vi "Create-server-channel.vi"(8 "error in (no error)":errorcluster, 11 "ModComm in":T1) -> (0 "error out":errorcluster, 2 "ServerChannel":refnum<queue>, 3 "ModComm out":T1)   [LabVIEW 2013, in "SLMServer.lvlib" / "SLMServer.lvclass"]
uses:
  SLMServer.lvclass
  Object-reference.ctl
  SA-SLMAPI/Sources/Message.lvclass
  SLMServer.lvclass/SLMServer.ctl
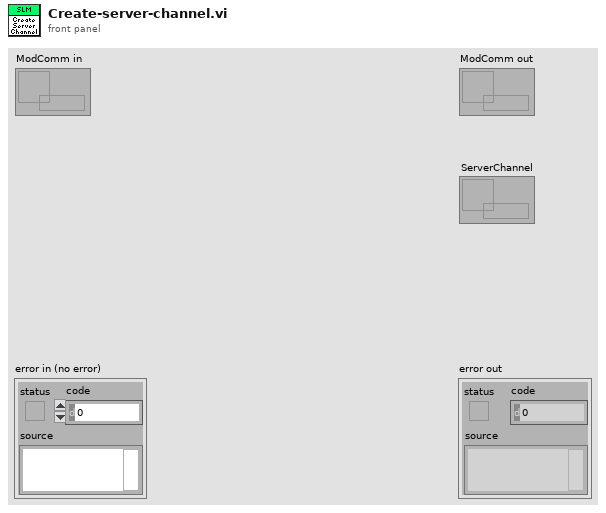
[diagram p1: front panel]
types:
  T1 = typedef "SLMServer.lvlib/SLMServer.lvclass/Object-reference.ctl" = refnum<data-value>
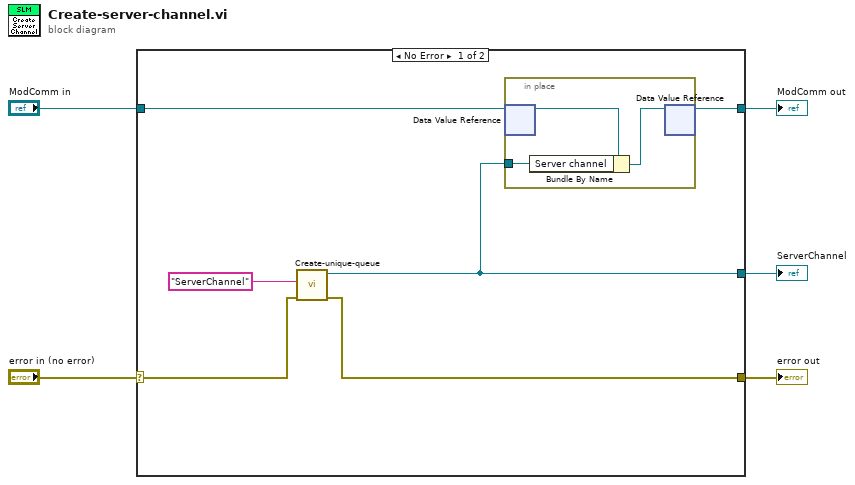
[diagram p0: block diagram]
diagram:
  n1 = case shown="No Error" "error in (no error)" {
    selector: "error in (no error)" -> [w11 w16]
    tunnel: [w10 w16] -> w4
    tunnel: [w8 w15] -> w2
    tunnel: "ModComm in" -> [w9 w15]
    tunnel: [w7 _] -> w1
    frame No Error {
      n2 = call "Create-unique-queue.vi"("error in (no error)"=w11, "Prefix"="ServerChannel" ("name (unnamed)")) -> ("error out"=w10:errorcluster, "Queue out"=w7:refnum<queue>)  [unwired: 7 in, 1 out]
      n3 = in-place {
        in-place-border: w7 -> [w12]
        n4 = in-place-dvr #1(w9) -> (w14:refnum<class "SLMServer.lvclass">)  [unwired: 1 out]
        n5 = Bundle By Name(cluster=w14, "Server channel"=w12) -> (w13:refnum<class "SLMServer.lvclass">)
        n6 = in-place-dvr #1(w13) -> (w8:T1)  [unwired: 1 out]
      }
    }
    frame Error {
    }
  }
  "error out" <- w4
  "ModComm out" <- w2
  "ServerChannel" <- w1
